vi "Slider Scale and Name Updater.vi"(8 "error in (no error)":errorcluster, 11 "Cluster In":T1) -> (0 "error out":errorcluster, 3 "Cluster Out":T1)   [LabVIEW 2018]
uses:
  Shared Controls/Range Updater.ctl
  Val Change Checker.vi
panel:
  in  "Boolean":bool
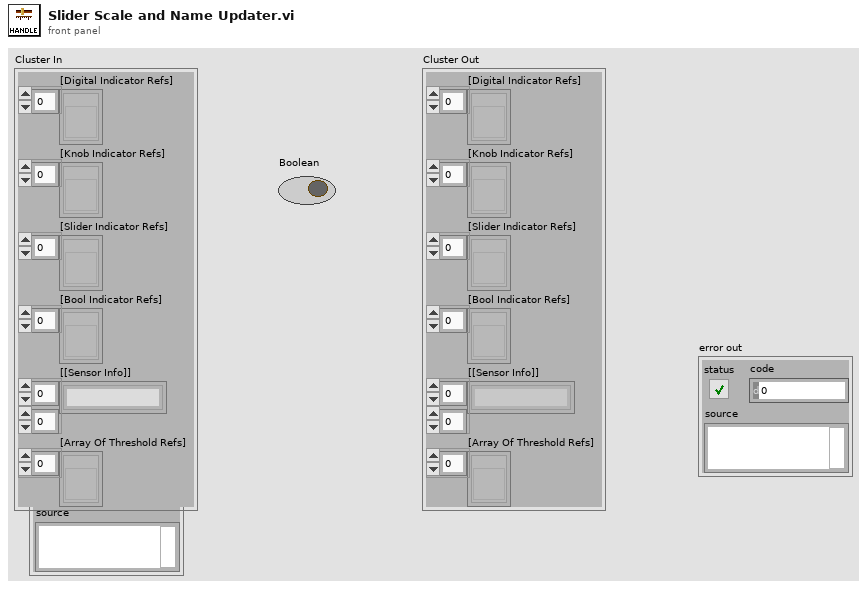
[diagram p1: front panel]
types:
  T1 = typedef "Range Updater.ctl" = cluster{"[Digital Indicator Refs]":refnum<vi>[], "[Knob Indicator Refs]":refnum<vi>[], "[Slider Indicator Refs]":refnum<vi>[], "[Bool Indicator Refs]":refnum<vi>[], "[[Sensor Info]]":string[][], "[Array Of Threshold Refs]":refnum<vi>[]}
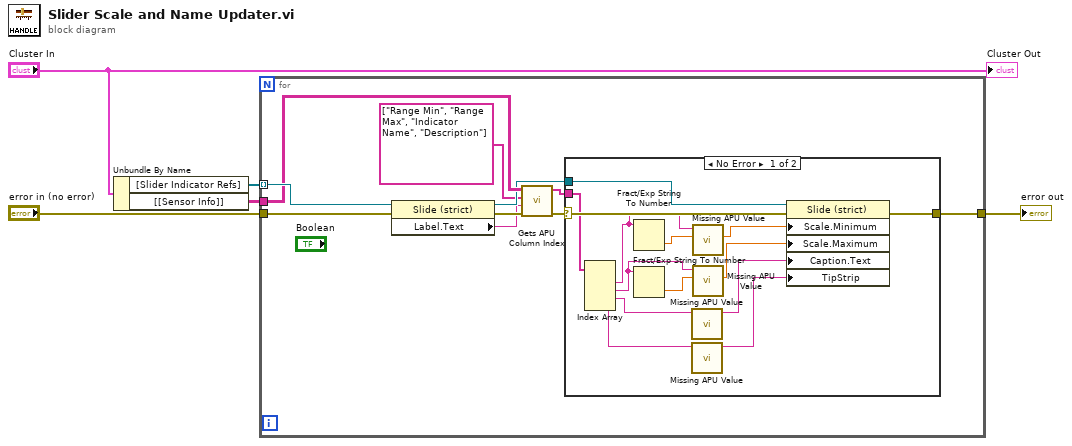
[diagram p0: block diagram]
diagram:
  n1 = Unbundle By Name("Cluster In") -> ("[Slider Indicator Refs]"=w4:refnum<vi>[], "[[Sensor Info]]"=w3:string[][])
  n2 = for {
    tunnel: w4 -> [w15] mode=indexing
    tunnel: "error in (no error)" -> [w14]
    tunnel: w3 -> [w11]
    tunnel: [w12] -> w2
    n3 = property class="Slide (strict)"(reference=w15, error in=w14) -> (reference out=w10:refnum<vi>, error out=w13:errorcluster, "Label.Text"=w6:string)
    n4 = call "Gets APU Column Index.vi"("error in (no error)"=w13, "Tag"=w6, "[Column Names]"=string[] ["Range Min", "Range Max", "Indicator Name", "Description"], "[[Array of Info]]"=w11) -> ("error out"=w9:errorcluster, "[Values out]"=w8:string[])  [unwired: 3 in, 3 out]
    n5 = case shown="No Error" w9 {
      selector: w9 -> [w29 w30]
      tunnel: [w28 w30] -> w12
      tunnel: w10 -> [w27 _]
      tunnel: w8 -> [w26 _]
      frame No Error {
        n6 = Index Array(array=w26) -> (element #1=w25:string, element #2=w23:string, element #3=w19:string, element #4=w17:string)  [unwired: 4 in]
        n7 = Fract/Exp String To Number(string=w25) -> (number=w21:dbl)  [unwired: 3 in, 1 out]
        n8 = Fract/Exp String To Number(string=w23) -> (number=w22:dbl)  [unwired: 3 in, 1 out]
        n9 = call "Missing APU Value.vi"("String In"=w19) -> ("String Out"=w18:string)  [unwired: 8 in, 2 out]
        n10 = call "Missing APU Value.vi"("String In"=w17) -> ("String Out"=w16:string)  [unwired: 8 in, 2 out]
        n11 = call "Missing APU Value.vi"("Num In"=w21, "String In"=w25) -> ("Num Out"=w24:dbl)  [unwired: 7 in, 2 out]
        n12 = call "Missing APU Value.vi"("Num In"=w22, "String In"=w23) -> ("Num Out"=w20:dbl)  [unwired: 7 in, 2 out]
        n13 = property class="Slide (strict)"(reference=w27, error in=w29, "Scale.Minimum"=w24, "Scale.Maximum"=w20, "Caption.Text"=w18, "TipStrip"=w16) -> (error out=w28:errorcluster)  [unwired: 1 out]
      }
      frame Error {
      }
    }
  }
  "error out" <- w2
  "Cluster Out" <- "Cluster In"
